vi "ClearCompileCache.vi"(8 "error in (no error)":errorcluster) -> (0 "error out":errorcluster)   [LabVIEW 2020, in "CICD.lvlib"]
uses:
  CICD.lvlib
  <vilib>/Wiresmith Technology/G CLI/CLI Class/CLI.lvclass
  <vilib>/Wiresmith Technology/G CLI/Argument Parser/Option Set Class/Option Set.lvclass
  <vilib>/Wiresmith Technology/G CLI/Argument Parser/Option Class/Option Configuration.ctl
  <vilib>/Wiresmith Technology/G CLI/Argument Parser/Option Class/Option.lvclass
  <vilib>/Wiresmith Technology/G CLI/Argument Parser/Option Class/Argument Type.ctl
  Helpers/Cache--enum.ctl
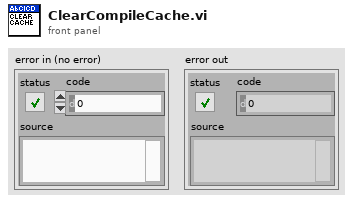
[diagram p1: front panel]
types:
  T1 = typedef "Option Parser.lvlib/Option.lvclass/Option Configuration.ctl" = cluster{"Option Type":T2, "Option Labels":string[], "Key":string, "Description":string, "Required":bool, "Default Value":string}
  T2 = typedef "Option Parser.lvlib/Option.lvclass/Argument Type.ctl" = enum16{"flag", "value"}
  T3 = typedef "CICD.lvlib/Cache--enum.ctl" = enum16{"All", "User", "AppBuilder"}
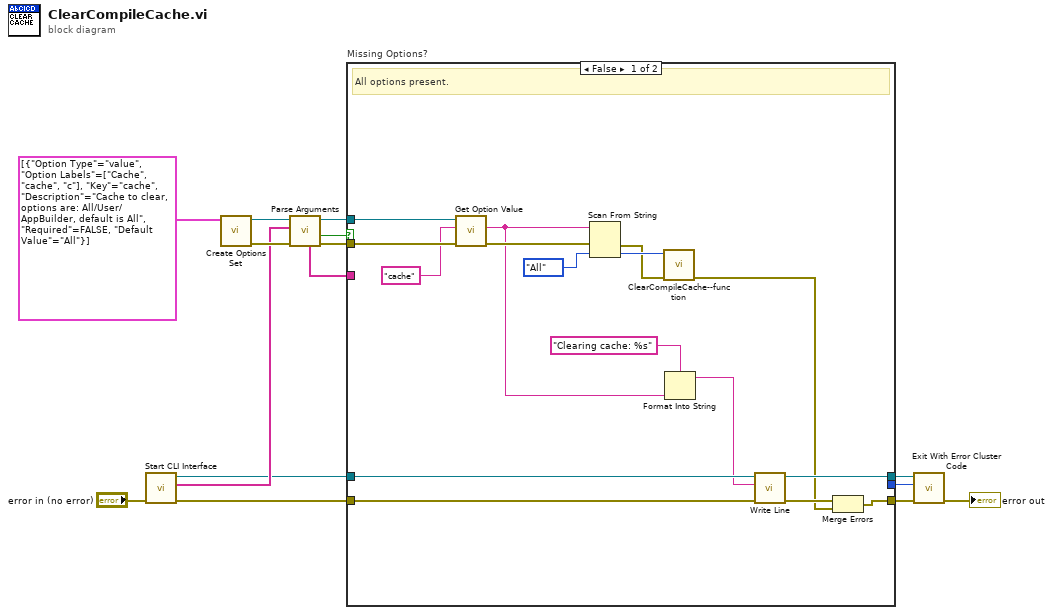
[diagram p0: block diagram]
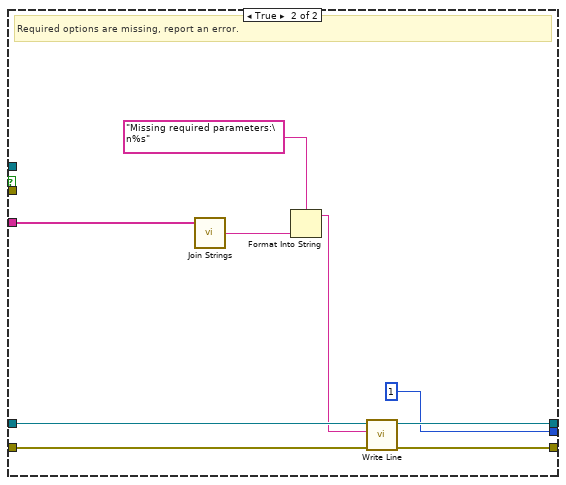
[diagram p2: hidden frame]
diagram:
  n1 = call <vilib>:"Start CLI Interface.vi"("error in (no error)"="error in (no error)") -> ("error out"=w7:errorcluster, "Custom Parameters"=w11:string[], "CLI out"=w6:refnum<class "CLI.lvclass">)  [unwired: 7 in, 1 out]
  n2 = call <vilib>:"Create Options Set.vi"("Options"=T1[] [{"Option Type"=enum."value", "Option Labels"=["Cache", "cache", "c"], "Key"="cache", "Description"="Cache to clear, options are: All/User/AppBuilder, default is All", "Required"=FALSE, "Default Value"="All"}]) -> ("error out"=w13:errorcluster, "Option Set out"=w14:refnum<class "Option Set.lvclass">)  [unwired: 9 in]
  n3 = call <vilib>:"Parse Arguments.vi"("error in (no error)"=w13, "Arguments"=w11, "Option Set in"=w14) -> ("error out"=w9:errorcluster, "Missing Options"=w10:bool, "Option Set out"=w1:refnum<class "Option Set.lvclass">, "Missing Option Keys"=w8:string[])  [unwired: 5 in]
  n4 = case "Missing Options?" shown="False" w10 {
    tunnel: w9 -> [w30 _]
    tunnel: w8 -> [_ w38]
    tunnel: w7 -> [w31 w37]
    tunnel: w6 -> [w22 w36]
    tunnel: [w20 w34] -> w5
    tunnel: [w21 w33] -> w3
    tunnel: [_ 1 ("No Error Code (0)")] -> w2
    tunnel: w1 -> [w29 _]
    frame False {
      # "All options present."
      n5 = call <vilib>:"Get Option Value.vi"("error in (no error)"=w30, "Option Key"="cache", "Option Set in"=w29) -> ("error out"=w24:errorcluster, "Value"=w18:string)  [unwired: 5 in, 2 out]
      n6 = Scan From String(input string=w18, error in=w24, default 1=Cache--enum."All" ("-Cache")) -> (error out=w25:errorcluster, output 1=w26:T3)  [unwired: 2 in, 2 out]
      n7 = call "ClearCompileCache--function.vi"("error in"=w25, "-Cache"=w26) -> ("error out"=w19:errorcluster)  [unwired: 9 in]
      n8 = Format Into String(format string="Clearing cache: %s", w18) -> (resulting string=w16:string)  [unwired: 2 in, 1 out]
      n9 = call <vilib>:"Write Line.vi"("error in (no error)"=w31, "Text to Write"=w16, "CLI in"=w22) -> ("error out"=w23:errorcluster, "CLI out"=w21:refnum<class "CLI.lvclass">)  [unwired: 7 in]
      n10 = Merge Errors(w23, w19) -> (w20:errorcluster)
    }
    frame True {
      # "Required options are missing, report an error."
      n11 = call <vilib>:"Join Strings.vi"("Strings In"=w38) -> ("String"=w39:string)  [unwired: 2 in]
      n12 = Format Into String(format string="Missing required parameters:\n%s" ("Text to Write"), w39) -> (resulting string=w35:string)  [unwired: 2 in, 1 out]
      n13 = call <vilib>:"Write Line.vi"("error in (no error)"=w37, "Text to Write"=w35, "CLI in"=w36) -> ("error out"=w34:errorcluster, "CLI out"=w33:refnum<class "CLI.lvclass">)  [unwired: 7 in]
    }
  }
  n14 = call <vilib>:"Exit With Error Cluster Code.vi"("error in (no error)"=w5, "No Error Code (0)"=w2, "CLI in"=w3) -> ("error out"=→"error out":errorcluster)  [unwired: 8 in]
